vi "GetPathsToIconEditorFilesInLVInstallationCLI.vi"() -> ()   [LabVIEW 2021]
uses:
  <vilib>/Wiresmith Technology/G CLI/CLI Class/CLI.lvclass
  <userlib>/_OpenG.lib/file/file.llb/openg_file.lvlib
panel:
  out "path":path
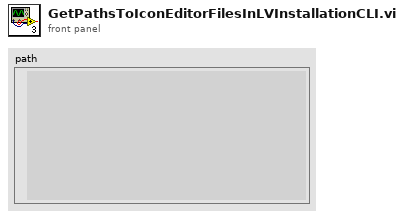
[diagram p1: front panel]
types:
  T1 = enum16{"open", "replace", "create", "open or create", "replace or create", "replace or create with confirmation"}
  T2 = enum32{"Invalid", "Standard", "Closed", "Hidden", "Minimized", "Maximized"}
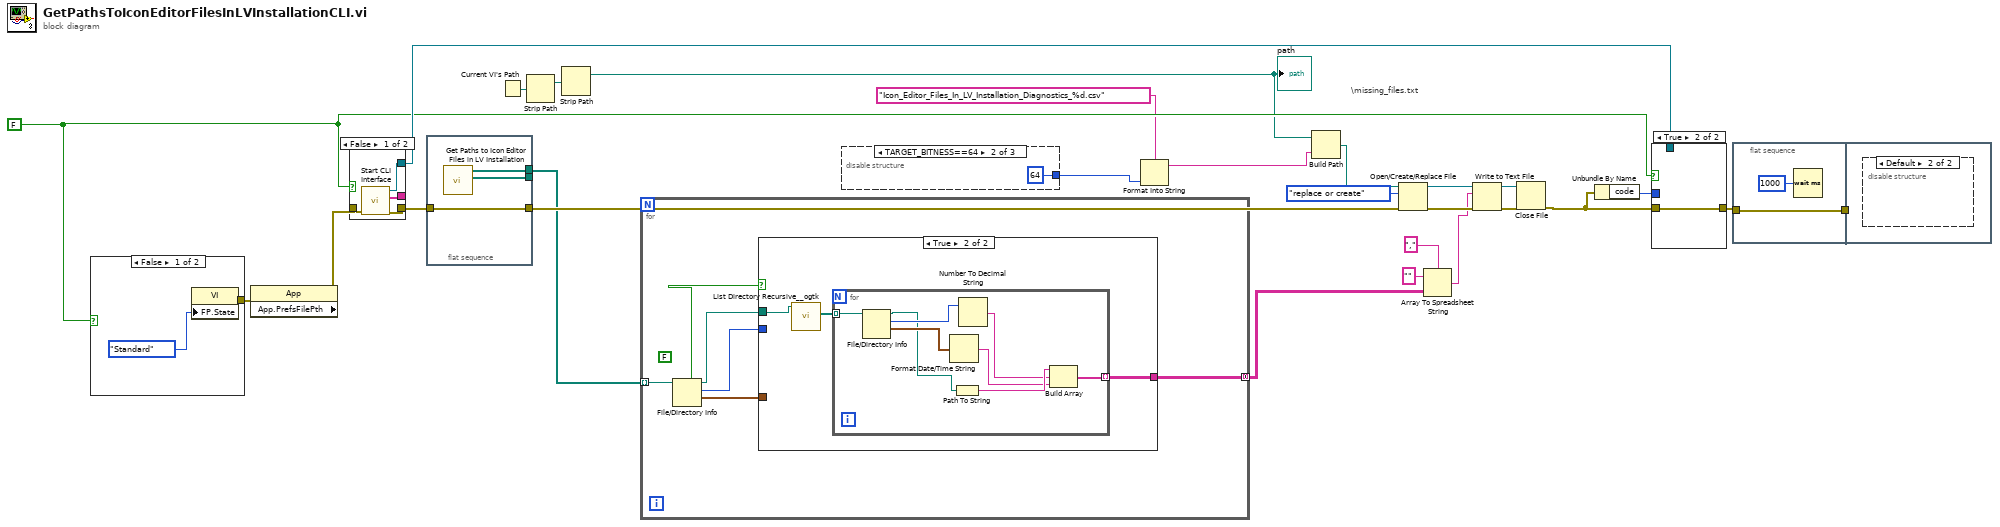
[diagram p0: block diagram]
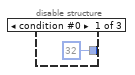
[diagram p2: hidden frame]
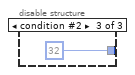
[diagram p3: hidden frame]
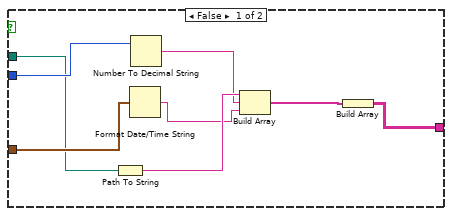
[diagram p4: hidden frame]
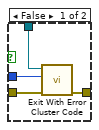
[diagram p5: hidden frame]
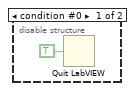
[diagram p8: hidden frame]
diagram:
  w21 = FALSE ("Debug")
  # "\\missing_files.txt"
  n1 = case shown="False" w21 {
    tunnel: [w28 _] -> w23
    frame False {
      n2 = property class="VI"("FP.State"=T2."Standard" ("Front Panel Window:State")) -> (error out=w28:errorcluster)  [unwired: 2 in, 1 out]
    }
    frame True {
    }
  }
  n3 = property class="App" props=["App.PrefsFilePth"](error in=w23) -> (error out=w22:errorcluster)  [unwired: 1 in, 2 out]
  n4 = case shown="False" w21 {
    tunnel: [w33 _] -> w27
    tunnel: w22 -> [w32 w34]
    tunnel: [w31 w34] -> w20
    tunnel: [w30 _] -> _
    frame False {
      n5 = call <vilib>:"Start CLI Interface.vi"("error in (no error)"=w32) -> ("error out"=w31:errorcluster, "Custom Parameters"=w30:string[], "CLI out"=w33:refnum<class "CLI.lvclass">)  [unwired: 7 in, 1 out]
    }
    frame True {
    }
  }
  n6 = flat-sequence {
    tunnel: w20 -> [w37]
    tunnel: [w37] -> w13
    tunnel: [w36] -> w9
    tunnel: [w35] -> _
    frame #0 {
      n7 = call "Get Paths to Icon Editor Files in LV Installation.vi"() -> ("relative paths"=w35:path[], "absolute paths"=w36:path[])  [unwired: 10 in]
    }
  }
  n8 = Current VI's Path() -> (path=w19:path)
  n9 = Strip Path(path=w19) -> (stripped path=w18:path)  [unwired: 1 out]
  n10 = Strip Path(path=w18) -> (stripped path=w11:path)  [unwired: 1 out]
  "path" <- w11
  n11 = for {
    tunnel: w9 -> [w43] mode=indexing
    tunnel: [w38] -> w4 mode=concatenating
    (unwired) FALSE ("directory")
    n12 = File/Directory Info(path=w43) -> (path out=w41:path, directory=w42:bool, size=w39:i64, last mod=w40:timestamp)  [unwired: 1 in, 3 out]
    n13 = case shown="True" w42 {
      tunnel: w41 -> [w49 w54]
      tunnel: w39 -> [w50 _]
      tunnel: w40 -> [w51 _]
      tunnel: [w47 w52] -> w38
      frame False {
        n14 = Path To String(path=w49) -> (string=w46:string)
        n15 = Format Date/Time String(seconds (now)=w51) -> (date/time string=w44:string)  [unwired: 2 in]
        n16 = Number To Decimal String(number=w50) -> (decimal integer string=w45:string)  [unwired: 1 in]
        n17 = Build Array(w46, w45, w44) -> (w48:string[])
        n18 = Build Array(w48) -> (w47:string[][])
      }
      frame True {
        n19 = call <userlib>:"List Directory Recursive__ogtk.vi"("Path"=w54) -> ("file paths"=w53:path[])  [unwired: 7 in, 3 out]
        n20 = for {
          tunnel: w53 -> [w62] mode=indexing
          tunnel: [w58] -> w52 mode=indexing
          n21 = File/Directory Info(path=w62) -> (path out=w59:path, size=w60:i64, last mod=w61:timestamp)  [unwired: 1 in, 4 out]
          n22 = Format Date/Time String(seconds (now)=w61) -> (date/time string=w55:string)  [unwired: 2 in]
          n23 = Path To String(path=w59) -> (string=w57:string)
          n24 = Number To Decimal String(number=w60) -> (decimal integer string=w56:string)  [unwired: 1 in]
          n25 = Build Array(w57, w56, w55) -> (w58:string[])
        }
      }
    }
  }
  n26 = disable-structure shown="TARGET_BITNESS==64" {
    disable-tunnel: [i64 32 ("size") i64 64 ("size") i64 32 ("size")] -> w3
    frame condition #0 {
    }
    frame condition #1 (active) {
    }
    frame condition #2 {
    }
  }
  n27 = Format Into String(format string="Icon_Editor_Files_In_LV_Installation_Diagnostics_%d.csv", w3) -> (resulting string=w1:string)  [unwired: 2 in, 1 out]
  n28 = Build Path(base path=w11, name or relative path=w1) -> (appended path=w10:path)
  n29 = Open/Create/Replace File(file path (use dialog)=w10, error in=w13, operation (0:open)=T1."replace or create") -> (refnum out=w14:refnum<file>, error out=w17:errorcluster)  [unwired: 3 in, 1 out]
  n30 = Array To Spreadsheet String(delimiter (Tab)=",", array=w4, 3:"" ("format string")) -> (spreadsheet string=w5:string)
  n31 = Write to Text File(file (use dialog)=w14, text=w5, error in=w17) -> (refnum out=w15:refnum<file>, error out=w16:errorcluster)  [unwired: 1 in, 1 out]
  n32 = Close File(refnum=w15, error in=w16) -> (error out=w12:errorcluster)  [unwired: 1 out]
  n33 = Unbundle By Name(w12) -> ("code"=w24:i32)
  n34 = case shown="True" w21 {
    tunnel: w27 -> [w69 _]
    tunnel: [w68 w70] -> w25
    tunnel: w24 -> [w67 _]
    tunnel: w12 -> [w66 w70]
    frame False {
      n35 = call <vilib>:"Exit With Error Cluster Code.vi"("error in (no error)"=w66, "No Error Code (0)"=w67, "CLI in"=w69) -> ("error out"=w68:errorcluster)  [unwired: 8 in]
    }
    frame True {
    }
  }
  n36 = flat-sequence {
    tunnel: w25 -> [w72]
    tunnel: [w72] -> w26
    tunnel: w26 -> [_]
    frame #0 {
      n37 = Wait (ms)(milliseconds to wait=u32 1000) -> ()  [unwired: 1 out]
    }
    frame #1 {
      n38 = disable-structure shown="Default" {
        frame condition #0 {
          n39 = Quit LabVIEW(quit? (T)=TRUE) -> ()
        }
        frame condition #1 (active) {
        }
      }
    }
  }
